vi "SaveModuleOffsets.vi"(10 "Write Swerve Offsets":bool, 11 "Swerve Voltages":dbl[](array[numeric])=[166.1, 59.2, 37.6, 148.1]) -> (3 "Swerve Offsets":dbl[](array[numeric])=[166.1, 59.2, 37.6, 148.1])   [LabVIEW 2018]
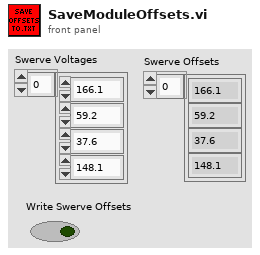
[diagram p1: front panel]
types:
  T1 = enum16{"open", "replace", "create", "open or create", "replace or create", "replace or create with confirmation"}
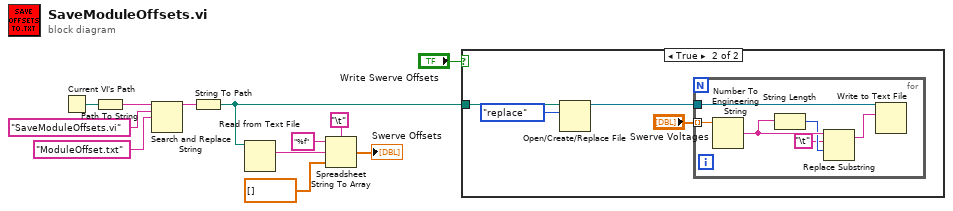
[diagram p0: block diagram]
diagram:
  n1 = Current VI's Path() -> (path=w6:path)
  n2 = Path To String(path=w6) -> (string=w5:string)
  n3 = Search and Replace String(input string=w5, search string="SaveModuleOffsets.vi" ("substring (\"\")"), replace string="ModuleOffset.txt" ("replace string (\"\")")) -> (result string=w2:string)  [unwired: 5 in, 3 out]
  n4 = String To Path(string=w2) -> (path=w1:path)
  n5 = Read from Text File(file (use dialog)=w1) -> (text=w11:string)  [unwired: 3 in, 3 out]
  n6 = Spreadsheet String To Array(delimiter (Tab)="\t", format string="%f", spreadsheet string=w11, array type (2D Dbl)=dbl[] []) -> (array=→"Swerve Offsets":dbl[])
  n7 = case shown="True" "Write Swerve Offsets" {
    tunnel: w1 -> [_ w14]
    frame False {
    }
    frame True {
      n8 = Open/Create/Replace File(file path (use dialog)=w14, operation (0:open)=T1."replace") -> (refnum out=w16:refnum<file>)  [unwired: 4 in, 2 out]
      n9 = for {
        tunnel: w16 -> [w22]
        tunnel: "Swerve Voltages" -> [w17] mode=indexing
        n10 = Number To Engineering String(4:w17) -> (0:w21:string)  [unwired: 3 in]
        n11 = String Length(string=w21) -> (length=w20:i32)
        n12 = Replace Substring(3:w20, 4:"\t", 5:w21) -> (1:w18:string)  [unwired: 1 in, 1 out]
        n13 = Write to Text File(file (use dialog)=w22, text=w18) -> ()  [unwired: 2 in, 3 out]
      }
    }
  }
